vi "IMU.vi"   [LabVIEW 2017]
uses:
  <vilib>/Platform/TimedLoop/XDataNode/timing_clust.ctl
  <vilib>/Platform/TimedLoop/XDataNode/nitl_modes.ctl
  <vilib>/Platform/TimedLoop/XDataNode/wakeup.ctl
  <vilib>/platform/TimedLoop/XDataNode/XDataNode.xnode
  <vilib>/Platform/TimedLoop/XDataNode/XDNodeRunTimeDep.lvlib
types:
  T1 = typedef "XDNodeRunTimeDep.lvlib/timing_clust.ctl" = cluster{"Expected End [f-1]":u64, "Actual End [f-1]":u64, "Finished Late? [f-1]":bool, "Expected End [i-1]":u64, "Actual End [i-1]":u64, "Finished Late? [i-1]":bool, "Expected Start [i]":u64, "Actual Start [i]":u64, "Expected Start [f]":u64, "Actual Start [f]":u64, "Source Name":string, "Structure Name":string, "Period":i64, "Deadline":i64, "Offset":i64, "Start":i64, "Priority":i32, "Timeout":i32, "Mode":T2, "Wakeup Reason":T3, "Error":errorcluster, "Source Type":string, "Secondary Source Type":string, "Global End Time":u64, "Global Start Time":u64, "Frame Duration":u64, "Iteration Duration":u64, "Assigned CPU":i32, "I/O Scan Engine Mode":u32}
  T2 = typedef "XDNodeRunTimeDep.lvlib/nitl_modes.ctl" = enum32{"No Change", "Process missed periods, maintain original phase", "Discard missed periods, maintain original phase", "Process missed periods, ignore original phase", "Discard missed periods, ignore original phase"}
  T3 = typedef "XDNodeRunTimeDep.lvlib/wakeup.ctl" = enum32{"Normal", "Aborted", "Asynchronous wakeup", "Timing source error", "Timed loop error", "Timeout"}
  T4 = typedef "ImuDevRef.ctl" = cluster{"I2CDevRef":T5, "Valid Cal File?":bool}
  T5 = typedef "WPI_I2CDevRef.ctl" = cluster{"DevStatus":errorcluster, "Device Address":u8, "Handle":i32, "I2C Bus":T6}
  T6 = typedef "i2c_bus.ctl" = enum16{"I2C On-Board", "I2C MXP", "Invalid"}
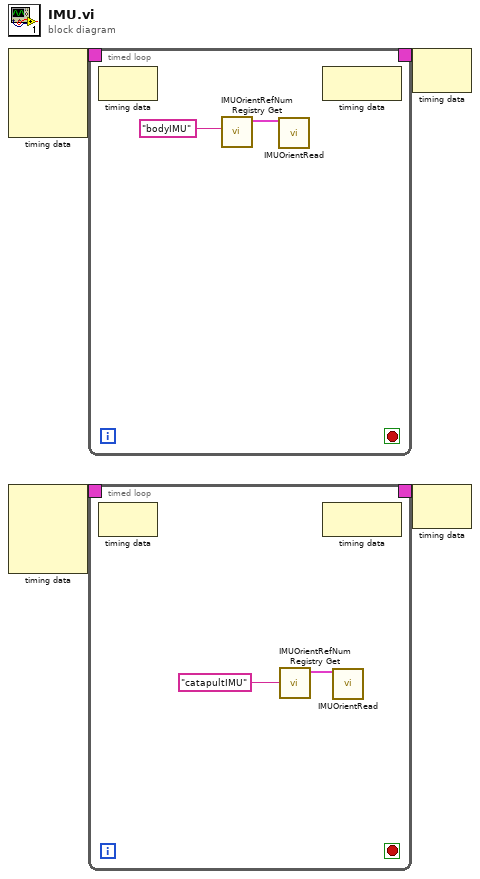
[diagram p0: block diagram]
diagram:
  n1 = node-c288() -> (w4:T1)  [unwired: 4 in]
  n2 = node-c288() -> (w2:T1)  [unwired: 4 in]
  n3 = timed-loop {
    timing: w4 -> [_]
    timing-out: [_] -> w3
    stop <- _ stop-if-true
    n4 = node-c288() -> ()  [unwired: 1 in, 1 out]
    n5 = call <userlib>:"IMUOrientRefNum Registry Get.vi"("refnum name"="bodyIMU") -> ("IMUDevRef out"=w5:T4)  [unwired: 9 in, 1 out]
    n6 = call <userlib>:"IMUOrientRead.vi"("IMU Dev Ref"=w5) -> ()  [unwired: 7 in, 8 out]
    n7 = node-c288() -> ()  [unwired: 1 in, 1 out]
  }
  n8 = timed-loop {
    timing: w2 -> [_]
    timing-out: [_] -> w1
    stop <- _ stop-if-true
    n9 = node-c288() -> ()  [unwired: 1 in, 1 out]
    n10 = call <userlib>:"IMUOrientRefNum Registry Get.vi"("refnum name"="catapultIMU") -> ("IMUDevRef out"=w9:T4)  [unwired: 9 in, 1 out]
    n11 = node-c288() -> ()  [unwired: 1 in, 1 out]
    n12 = call <userlib>:"IMUOrientRead.vi"("IMU Dev Ref"=w9) -> ()  [unwired: 7 in, 8 out]
  }
  n13 = node-c288(w3) -> ()  [unwired: 1 out]
  n14 = node-c288(w1) -> ()  [unwired: 1 out]
